vi "Union Unified Msg Set.vi"(11 "Base Actor in":refnum<class "Base Actor.lvclass">) -> (2 "Unified Msg Set":T1)   [LabVIEW 2020, in "jettl.lvlib" / "Actor.lvlib" / "Base Actor.lvclass"]
uses:
  Base Actor.lvclass
  Msg Set.ctl
  Msg/Msg.lvclass
  Base Actor.lvclass/Base Actor.ctl
  Actor.lvlib
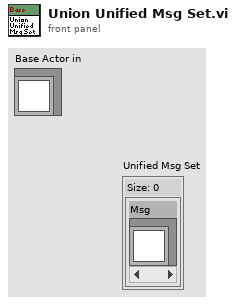
[diagram p1: front panel]
types:
  T1 = typedef "jettl.lvlib/Actor.lvlib/Msg Set.ctl" = set{refnum<class "Msg.lvclass">}
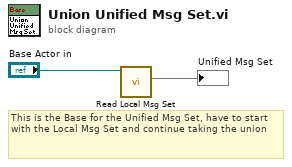
[diagram p0: block diagram]
diagram:
  # "This is the Base for the Unified Msg Set, have to start with the Local Msg Set and continue taking the union"
  n1 = call-dynamic "Read Local Msg Set.vi"("Base Actor in"="Base Actor in") -> ("Local Msg Set"=→"Unified Msg Set":T1)  [unwired: 10 in]
